vi "Aquire Data.vi"(8 "error in (no error)":errorcluster, 10 "Aqusition Time (s)":dbl, 11 "DAQ Process in":refnum<class "DAQ Process.lvclass">) -> (0 "error out":errorcluster, 3 "DAQ Process out":refnum<class "DAQ Process.lvclass">)   [LabVIEW 2022 SP3, in "DAQ Process.lvlib" / "DAQ Process.lvclass"]
uses:
  DAQ Process.lvclass
  DAQ Data/AIDAQ Data.ctl
  DAQ Process.lvclass/DAQ Process.ctl
  XY Stage/Process Actor/Process Framework/Process State Data/Process State Data.lvclass/Process State Data.ctl
  DAQ Data/DAQ Data.lvclass/DAQ Data.ctl
  XY Stage/Process Actor/Process Framework/Process State Data/Accessor/Read Abort.vi
  DAQ Data/Write AI Data.vi
  DAQ Data/Write appended array.vi
  AI Driver/AI Driver.lvclass
  XY Stage/Process Actor/Process Framework/Process State Data/Process State Data.lvclass
  DAQ Data/DAQ Data.lvclass
  DAQ Data/AI Daq Data.lvlib
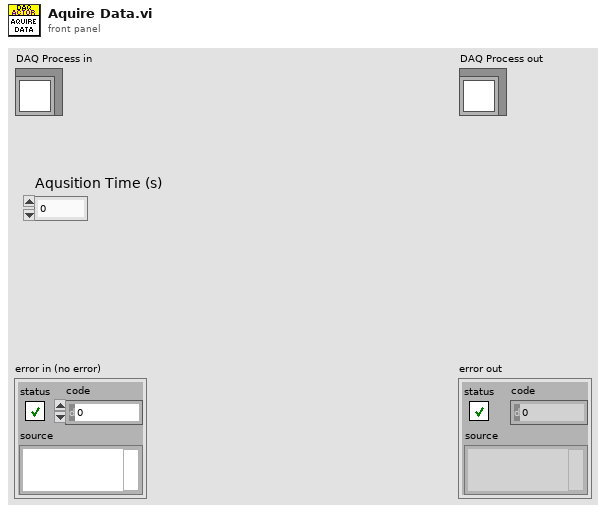
[diagram p1: front panel]
types:
  T1 = typedef "AI Daq Data.lvlib/AIDAQ Data.ctl" = cluster{"Time Stamp":timestamp, "AI":dbl}
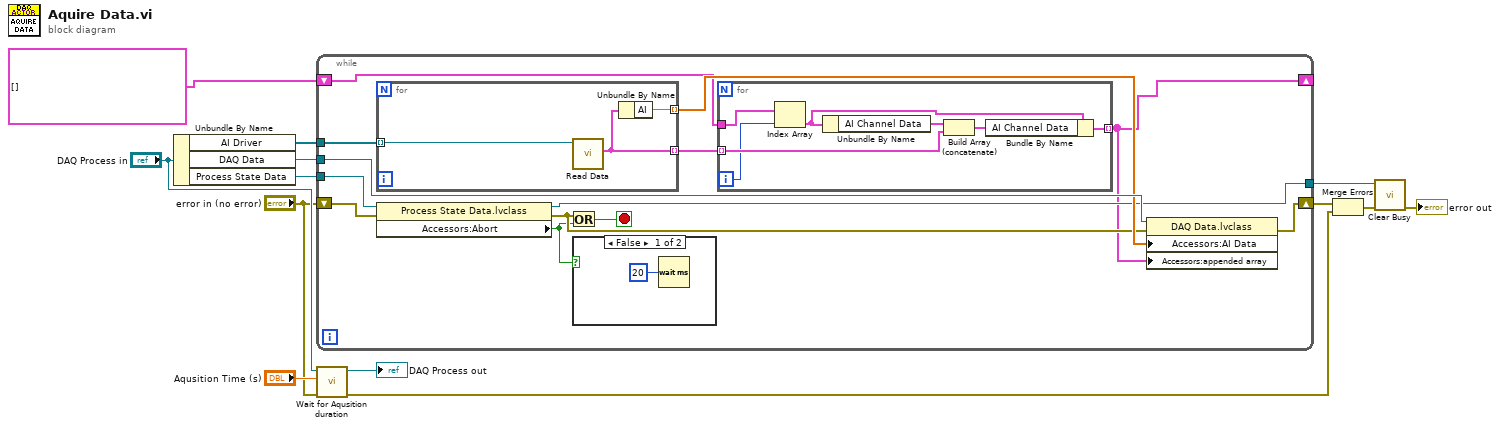
[diagram p0: block diagram]
diagram:
  n1 = Unbundle By Name("DAQ Process in") -> ("AI Driver"=w11:refnum<class "AI Driver.lvclass">[], "DAQ Data"=w10:refnum<data-value>, "Process State Data"=w9:refnum<data-value>)
  n2 = while {
    tunnel: w11 -> [w26]
    tunnel: w10 -> [w25]
    shift-right: [w14] -> _
    shift-left: cluster{"AI Channel Data":T1[]}[] [] ("Cluster") -> [w22]
    tunnel: w9 -> [w21]
    shift-right: [w19] -> w4
    shift-left: "error in (no error)" -> [w20]
    tunnel: [w15] -> w6
    stop <- w16 stop-if-true
    n3 = for {
      tunnel: w26 -> [w37] mode=indexing
      tunnel: [w36] -> w23 mode=indexing
      tunnel: [w35] -> w24 mode=indexing
      n4 = call-dynamic "Read Data.vi"("AI Driver in"=w37) -> ("Daq Data"=w36:T1)  [unwired: 8 in, 2 out]
      n5 = Unbundle By Name(w36) -> ("AI"=w35:dbl)
    }
    n6 = property class="Process State Data.lvclass"(reference=w21, error in=w20) -> (reference out=w15:refnum<data-value>, error out=w18:errorcluster, "Accessors:Abort"=w17:bool)
    n7 = Or(x=w18, y=w17) -> (x .or. y?=w16:bool)
    n8 = case shown="False" w17 {
      frame False {
        n9 = Wait (ms)(milliseconds to wait=u32 20) -> ()  [unwired: 1 out]
      }
      frame True {
      }
    }
    n10 = for {
      tunnel: w23 -> [w33] mode=indexing
      tunnel: w22 -> [w29]
      tunnel: [w31] -> w14 mode=indexing
      i -> [w30]
      n11 = Index Array(array=w29, index=w30) -> (element=w28:cluster{"AI Channel Data":T1[]})
      n12 = Unbundle By Name(w28) -> ("AI Channel Data"=w34:T1[])
      n13 = Build Array (concatenate)(w34, w33) -> (w32:T1[])
      n14 = Bundle By Name(cluster=w28, "AI Channel Data"=w32) -> (w31:cluster{"AI Channel Data":T1[]})
    }
    n15 = property class="DAQ Data.lvclass"(reference=w25, error in=w18, "Accessors:AI Data"=w24, "Accessors:appended array"=w14) -> (error out=w19:errorcluster)  [unwired: 1 out]
  }
  n16 = call "Wait for Aqusition duration.vi"("error in (no error)"="error in (no error)", "Aqusition Time (s)"="Aqusition Time (s)", "DAQ Process in"="DAQ Process in") -> ("error out"=w5:errorcluster, "DAQ Process\\"=→"DAQ Process out":refnum<class "DAQ Process.lvclass">)  [unwired: 7 in]
  n17 = Merge Errors(w4, w5) -> (w3:errorcluster)
  n18 = call "Clear Busy.vi"("error in (no error)"=w3, "Process State"=w6) -> ("error out"=→"error out":errorcluster)  [unwired: 8 in, 1 out]
